vi "Toggle Relay.vi"(8 "error in":errorcluster, 9 "Relay State":bool, 10 "Relay Name":string, 11 "SwitchMatrix in":refnum<class "SwitchMatrix.lvclass">) -> (0 "error out":errorcluster, 3 "SwitchMatrix out":refnum<class "SwitchMatrix.lvclass">)   [LabVIEW 2019, in "SwitchMatrix.lvlib" / "SwitchMatrix.lvclass"]
doc: "Set one relay state to either on or off."
uses:
  Library/SwitchMatrix.lvclass
  C:/Users/Public/Documents/Development/builds/Instruments/Instruments.lvlibp/Library/Instruments.lvclass
  builds/Instruments/Instruments.lvlibp/Private/Polymorphic/Special/Event from Boolean.vi
  builds/Instruments/Instruments.lvlibp/Accessors/Command with Logging.vi
  builds/Instruments/Instruments.lvlibp/Library/Instruments.lvclass
  builds/Engine/Engine.lvlibp/Project/Engine.lvclass
  builds/Instruments/Instruments.lvlibp
  C:/Users/Public/Documents/Development/builds/Engine/Engine.lvlibp/Project/Engine.lvclass
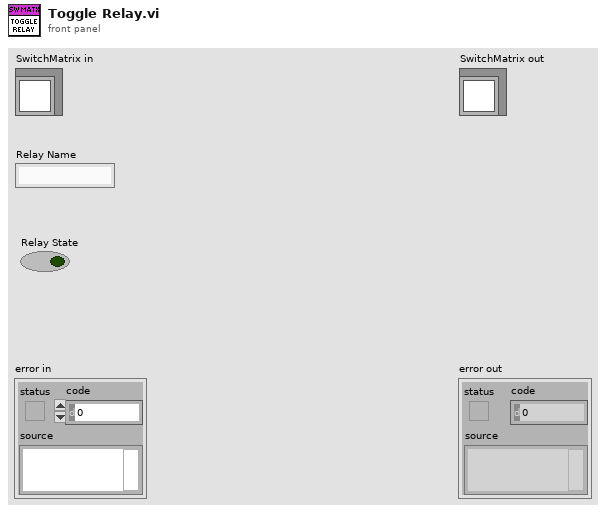
[diagram p1: front panel]
types:
  T1 = cluster{"Timestamp":timestamp, "Description":string, "Data":string}
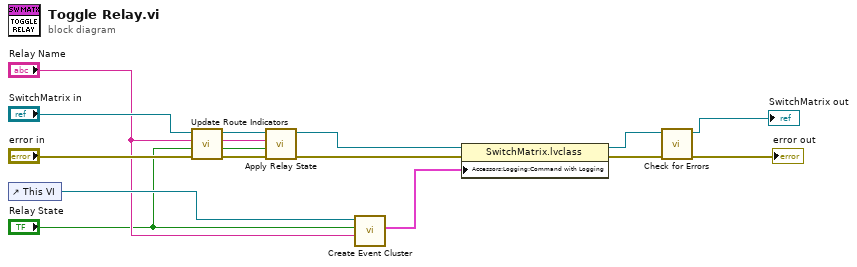
[diagram p0: block diagram]
diagram:
  n1 = control-ref of="This VI"() -> (w16:refnum<vi>)
  n2 = call "Update Route Indicators.vi"("error in"="error in", "State in"="Relay State", "Name in"="Relay Name", "SwitchMatrix in"="SwitchMatrix in") -> ("error out"=w12:errorcluster, "State out"=w9:bool, "Name out"=w10:string, "SwitchMatrix out"=w11:refnum<class "SwitchMatrix.lvclass">)  [unwired: 4 in]
  n3 = call "Apply Relay State.vi"("error in"=w12, "State"=w9, "Name"=w10, "SwitchMatrix in"=w11) -> ("error out"=w14:errorcluster, "SwitchMatrix out"=w13:refnum<class "SwitchMatrix.lvclass">)  [unwired: 6 in]
  n4 = call-poly "Create Event Cluster.vi"("Name"="Relay Name", "Value"="Relay State", "VI Refnum"=w16) -> ("Event Data"=w15:T1)  [unwired: 8 in]
  n5 = property class="SwitchMatrix.lvclass"(reference=w13, error in=w14, "Accessors:Logging:Command with Logging"=w15) -> (reference out=w2:refnum<class "SwitchMatrix.lvclass">, error out=w4:errorcluster)
  n6 = call "Check for Errors.vi"("error in"=w4, "Engine in"=w2) -> ("error out"=→"error out":errorcluster, "Engine out"=→"SwitchMatrix out":refnum<class "SwitchMatrix.lvclass">)  [unwired: 8 in]
